vi "Write TaskConfig.vi"(8 "error in (no error)":errorcluster, 10 "TaskConfig":T1={"Drive"=enum."NI_DAQmx", "TaskType"=enum."AI", "PhysicalChannels"="", "SampleRateConfiguration"={"SampleRate"=0.0, "SamplesPerChannel"=0, "SamplesPerRead"=0, "SampleMode"=10123, "Clock Source"="OnboardClock"}, "ChannelConfig"="", "Enable"=FALSE} {"SampleRateConfiguration"."SampleMode" items=["Finite Samples"=10178, "Continuous Samples"=10123, "Hardware Timed Single Point"=12522]}, 11 "Linear_Task in":refnum<class "Linear_Task.lvclass">) -> (0 "error out":errorcluster, 3 "Linear_Task out":refnum<class "Linear_Task.lvclass">)   [LabVIEW 2025, in "Linear_Task.lvlib" / "Linear_Task.lvclass"]
uses:
  Linear_Task.lvclass
  Linear_Task.lvclass/Linear_Task.ctl
  164c0d0e-bd4a-48b5-84b4-1267b11fb074.vi
  DAQ_Module/DAQ_Module/DAQ_Module/DAQ_Linear_Task_Config.ctl
  DAQ_Module/DAQ_Module/DAQ_Module/DAQ_Module.lvclass
  Task_Abstr/Task_Abstr/Task_Abstr.lvclass
  DAQ_Module/DAQ_Module/DAQ_Module/DAQ_Task_Type.ctl
  DAQ_Module/DAQ_Module/DAQ_Module/DAQ_Task_Config.ctl
  DAQ_Module/DAQ_Module/DAQ_Module/DAQ_HW_Type.ctl
  DAQ_Module/DAQ_Module/DAQ_Module/DAQ_SampleRateConfig.ctl
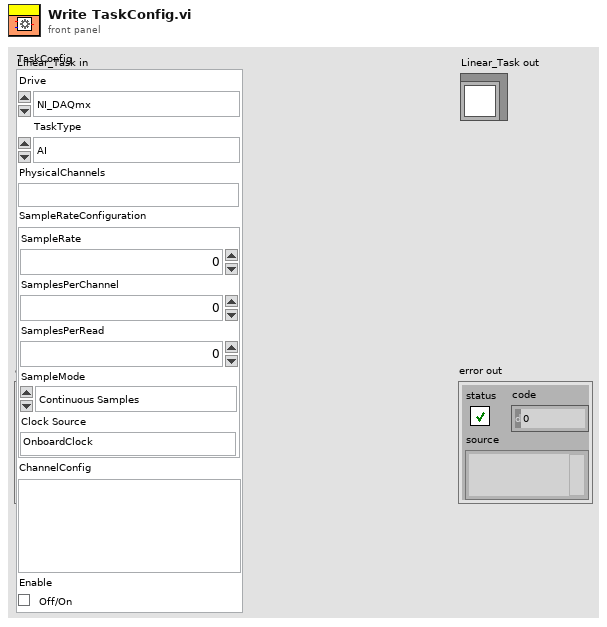
[diagram p1: front panel]
types:
  T1 = typedef "DAQ_Module.lvlib/DAQ_Module.lvclass/DAQ_Task_Config.ctl" = cluster{"Drive":T2, "TaskType":T3, "PhysicalChannels":string, "SampleRateConfiguration":T4, "ChannelConfig":string, "Enable":bool}
  T2 = typedef "DAQ_Module.lvlib/DAQ_Module.lvclass/DAQ_HW_Type.ctl" = enum16{"NI_DAQmx", "Simulated_DAQ"}
  T3 = typedef "DAQ_Module.lvlib/DAQ_Module.lvclass/DAQ_Task_Type.ctl" = enum16{"AI", "Linear", "Angular", "AO"}
  T4 = typedef "DAQ_Module.lvlib/DAQ_Module.lvclass/DAQ_SampleRateConfig.ctl" = cluster{"SampleRate":dbl, "SamplesPerChannel":u32, "SamplesPerRead":i32, "SampleMode":i32, "Clock Source":string}
  T5 = typedef "DAQ_Module.lvlib/DAQ_Module.lvclass/DAQ_Linear_Task_Config.ctl" = cluster{"decoding type":i32, "units":i32, "distance per pulse":dbl, "initial position":dbl, "z index enable":bool, "z index value":dbl, "z index phase":i32}
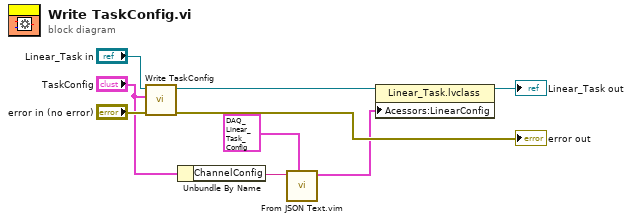
[diagram p0: block diagram]
diagram:
  n1 = call-parent "Write TaskConfig.vi"("error in (no error)"="error in (no error)", "TaskConfig"="TaskConfig", "Task_Abstr in"="Linear_Task in") -> ("error out"=→"error out":errorcluster, "Task_Abstr out"=w8:refnum<class "Linear_Task.lvclass">)  [unwired: 7 in]
  n2 = Unbundle By Name("TaskConfig") -> ("ChannelConfig"=w5:string)
  n3 = call "From JSON Text.vim"("Data Type and Default Value"=T5 {"decoding type"=10092, "units"=10219, "distance per pulse"=0.001, "initial position"=0.0, "z index enable"=FALSE, "z index value"=0.0, "z index phase"=10040} ("LinearConfig"), "JSON"=w5) -> ("Data out"=w1:T5)  [unwired: 8 in, 1 out]
  n4 = property class="Linear_Task.lvclass"(reference=w8, "Acessors:LinearConfig"=w1) -> (reference out=→"Linear_Task out":refnum<class "Linear_Task.lvclass">)  [unwired: 1 in, 1 out]
